vi "Record Data.vi"(8 "error in (no error)":errorcluster, 10 "Number of samples":i32=-1, 11 "Pulse Driver in":refnum<class "Pulse Driver.lvclass">) -> (0 "error out":errorcluster, 3 "Pulse Driver out":refnum<class "Pulse Driver.lvclass">)   [LabVIEW 2015, in "Pulse Driver.lvclass"]
uses:
  Pulse Driver.lvclass
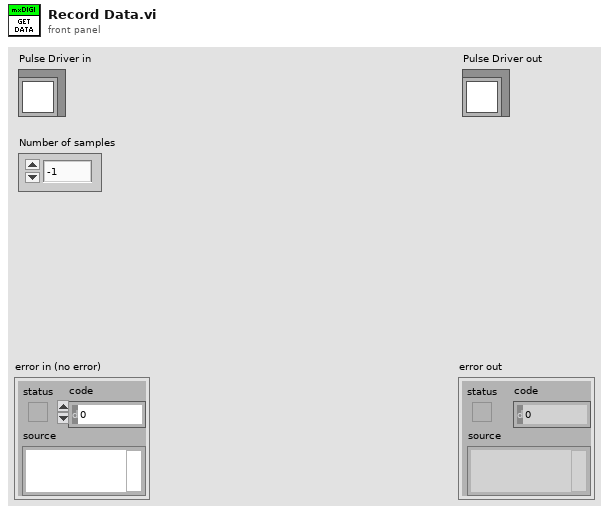
[diagram p1: front panel]
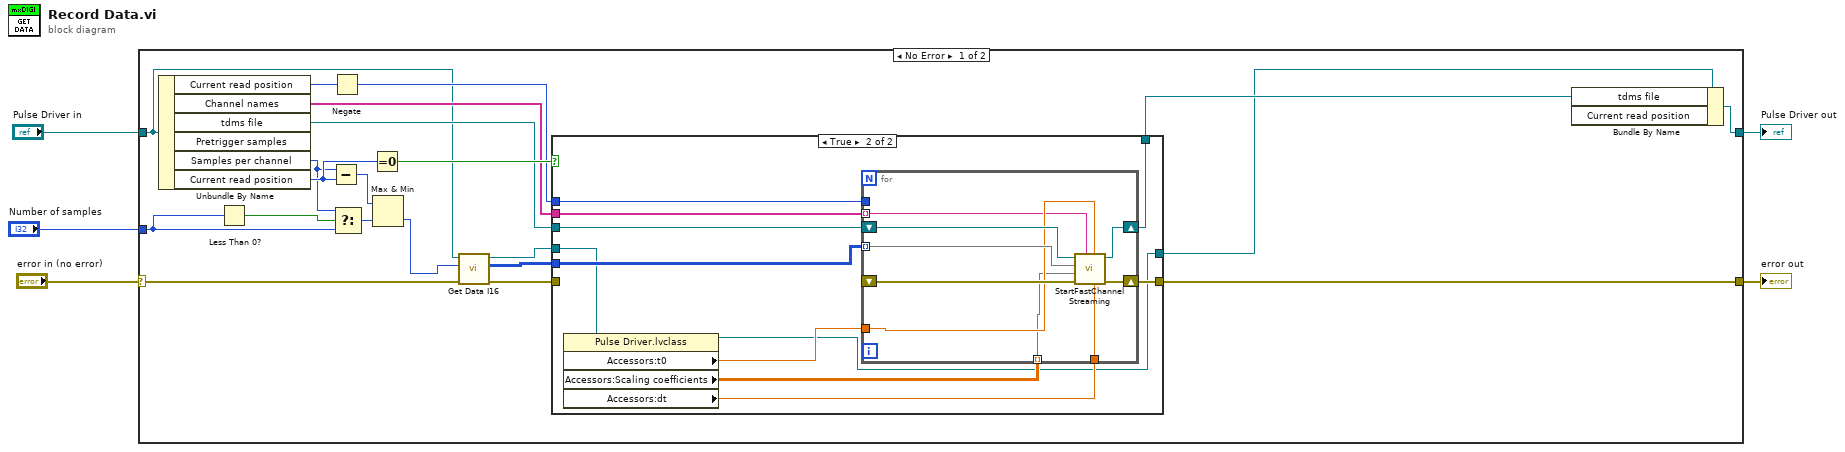
[diagram p0: block diagram]
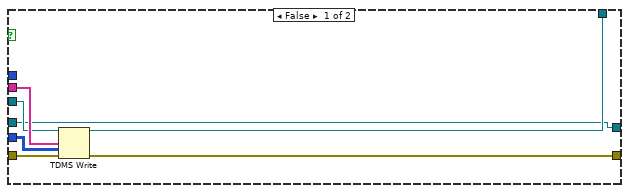
[diagram p2: hidden frame]
diagram:
  n1 = case shown="No Error" "error in (no error)" {
    selector: "error in (no error)" -> [w16 w55]
    tunnel: [w14 w55] -> w4
    tunnel: [w15 w54] -> w2
    tunnel: "Pulse Driver in" -> [w7 w54]
    tunnel: "Number of samples" -> [w11 _]
    frame No Error {
      n2 = Unbundle By Name(w7) -> ("Current read position"=w19:i32, "Channel names"=w18:string[], "tdms file"=w17:refnum<k34>, "Samples per channel"=w12:i32, "Current read position"=w23:i32)  [unwired: 1 out]
      n3 = Less Than 0?(x=w11) -> (x < 0?=w13:bool)
      n4 = Subtract(x=w12, y=w23) -> (x-y=w26:i32)
      n5 = Negate(x=w19) -> (-x=w20:i32)
      n6 = Select(t=w12, s=w13, f=w11) -> (s? t:f=w10:i32)
      n7 = Equal To 0?(x=w23) -> (x = 0?=w22:bool)
      n8 = Max & Min(x=w26, y=w10) -> (min(x,y)=w9:i32)  [unwired: 1 out]
      n9 = call-dynamic "Get Data I16.vi"("error in (no error)"=w16, "Number of samples per channel"=w9, "Pulse Driver in"=w7) -> ("error out"=w24:errorcluster, "Data out"=w21:i16[][], "Pulse Driver out"=w25:refnum<class "Pulse Driver.lvclass">)  [unwired: 6 in]
      n10 = case shown="True" w22 {
        tunnel: w25 -> [w27 w39]
        tunnel: w24 -> [w30 _]
        tunnel: w21 -> [w33 w44]
        tunnel: w20 -> [_ w43]
        tunnel: w18 -> [w32 w42]
        tunnel: w17 -> [w31 w41]
        tunnel: [w29 w40] -> w14
        tunnel: [w28 w36] -> w8
        tunnel: [w27 w34] -> w6
        frame False {
          n11 = TDMS Write(0:w31, 7:w32, 9:w33, 11:w30) -> (4:w28:refnum<k34>, 15:w29:errorcluster)  [unwired: 2 in, 2 out]
        }
        frame True {
          n12 = property class="Pulse Driver.lvclass"(reference=w39) -> (reference out=w34:refnum<class "Pulse Driver.lvclass">, "Accessors:t0"=w38:dbl, "Accessors:Scaling coefficients"=w35:dbl[][], "Accessors:dt"=w37:dbl)  [unwired: 1 in, 1 out]
          n13 = for {
            tunnel: w44 -> [w53] mode=indexing
            tunnel: w38 -> [w48]
            tunnel: w43 -> [_]
            tunnel: w42 -> [w46] mode=indexing
            shift-right: [w51] -> w36
            shift-left: w41 -> [w52]
            shift-right: [w49] -> w40
            shift-left: _ -> [w50]
            tunnel: w37 -> [w47]
            tunnel: w35 -> [w45] mode=indexing
            n14 = call "StartFastChannelStreaming.vi"("dt"=w47, "t0"=w48, "channel name(s) in (Untitled)"=w46, "error in (no error)"=w50, "Scaling coefficients"=w45, "Data"=w53, "tdms file"=w52) -> ("error out"=w49:errorcluster, "tdms file out"=w51:refnum<k34>)  [unwired: 3 in]
          }
        }
      }
      n15 = Bundle By Name(cluster=w6, "tdms file"=w8) -> (w15:refnum<class "Pulse Driver.lvclass">)  [unwired: 1 in]
    }
    frame Error {
    }
  }
  "error out" <- w4
  "Pulse Driver out" <- w2
